vi "Set Wheel Parameter by Name.vi"(8 "error in (no error)":errorcluster, 9 "parameter value":variant, 10 "parameter name":string, 11 "wheel in":refnum<class "NI_Robotics_Wheel.lvclass">) -> (0 "error out":errorcluster, 1 "set?":bool, 3 "wheel out":refnum<class "NI_Robotics_Wheel.lvclass">)   [LabVIEW 2017, in "NI_Robotics_Wheel.lvclass"]
uses:
  <vilib>/robotics/Steering/Wheel/NI_Robotics_Wheel.lvclass
  <vilib>/robotics/Steering/Wheel/NI_Robotics_Wheel.lvclass/NI_Robotics_Wheel.ctl
  <vilib>/robotics/Steering/Wheel/Rotation Direction.ctl
  <vilib>/robotics/Actuation/Motor Communication/NI_Robotics_Motor Communication.lvclass
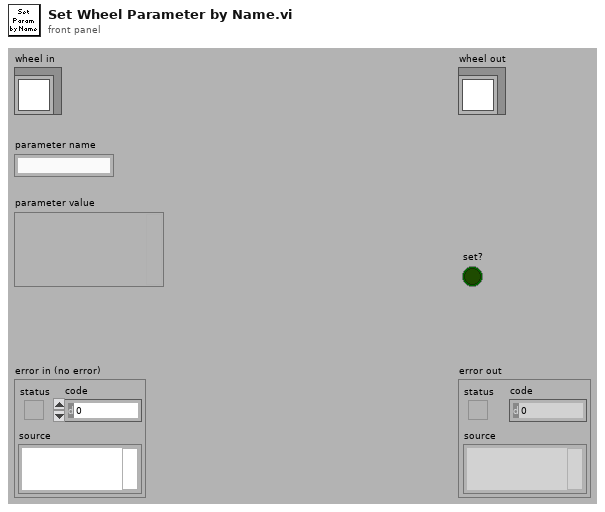
[diagram p1: front panel]
types:
  T1 = typedef "NI_Robotics_Wheel.lvclass/Rotation Direction.ctl" = u16
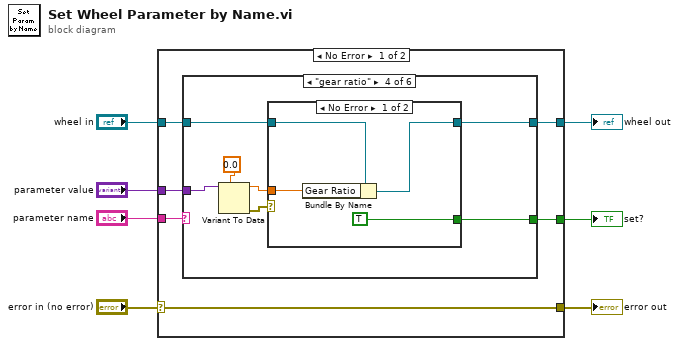
[diagram p0: block diagram]
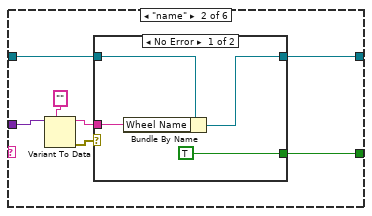
[diagram p3: hidden frame]
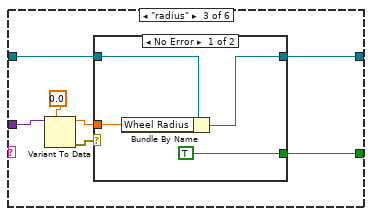
[diagram p5: hidden frame]
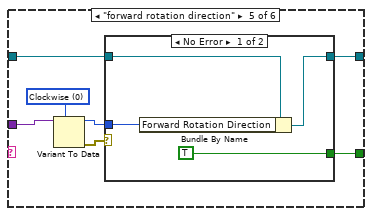
[diagram p8: hidden frame]
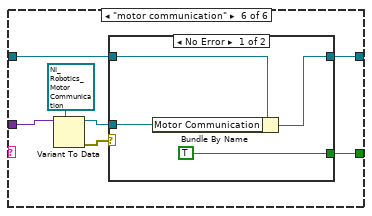
[diagram p10: hidden frame]
diagram:
  n1 = case shown="No Error" "error in (no error)" {
    selector: "error in (no error)" -> [w8 w76]
    tunnel: [w8 w76] -> w6
    tunnel: [w11 w75] -> w4
    tunnel: "wheel in" -> [w13 w75]
    tunnel: "parameter name" -> [w12 _]
    tunnel: "parameter value" -> [w10 _]
    tunnel: [w9 _] -> w1
    frame No Error {
      n2 = case shown="\"gear ratio\"" w12 {
        tunnel: w13 -> [w14 w17 w29 w41 w54 w66]
        tunnel: [w14 w16 w28 w40 w53 w65] -> w11
        tunnel: w10 -> [_ w21 w33 w45 w57 w69]
        tunnel: [_ w15 w27 w39 w52 w64] -> w9
        frame Default {
        }
        frame "name" {
          n3 = Variant To Data(type="", Variant=w21) -> (data=w18:string, error out=w19:errorcluster)  [unwired: 1 in]
          n4 = case shown="No Error" w19 {
            tunnel: w18 -> [w24 _]
            tunnel: w17 -> [w25 w26]
            tunnel: [w23 w26] -> w16
            tunnel: [TRUE _] -> w15
            frame No Error {
              n5 = Bundle By Name(cluster=w25, "Wheel Name"=w24) -> (w23:refnum<class "NI_Robotics_Wheel.lvclass">)
            }
            frame Error {
            }
          }
        }
        frame "radius" {
          n6 = Variant To Data(type=0.0, Variant=w33) -> (data=w30:dbl, error out=w31:errorcluster)  [unwired: 1 in]
          n7 = case shown="No Error" w31 {
            tunnel: w30 -> [w36 _]
            tunnel: w29 -> [w37 w38]
            tunnel: [w35 w38] -> w28
            tunnel: [TRUE _] -> w27
            frame No Error {
              n8 = Bundle By Name(cluster=w37, "Wheel Radius"=w36) -> (w35:refnum<class "NI_Robotics_Wheel.lvclass">)
            }
            frame Error {
            }
          }
        }
        frame "gear ratio" {
          n9 = Variant To Data(type=0.0, Variant=w45) -> (data=w42:dbl, error out=w43:errorcluster)  [unwired: 1 in]
          n10 = case shown="No Error" w43 {
            tunnel: w42 -> [w48 _]
            tunnel: w41 -> [w49 w50]
            tunnel: [w47 w50] -> w40
            tunnel: [TRUE _] -> w39
            frame No Error {
              n11 = Bundle By Name(cluster=w49, "Gear Ratio"=w48) -> (w47:refnum<class "NI_Robotics_Wheel.lvclass">)
            }
            frame Error {
            }
          }
        }
        frame "forward rotation direction" {
          w51 = T1 0 items=["Clockwise", "Counterclockwise"] ("Forward Rotation Direction")
          n12 = Variant To Data(type=w51, Variant=w57) -> (data=w55:T1, error out=w56:errorcluster)  [unwired: 1 in]
          n13 = case shown="No Error" w56 {
            tunnel: w55 -> [w58 _]
            tunnel: w54 -> [w61 w62]
            tunnel: [w60 w62] -> w53
            tunnel: [TRUE _] -> w52
            frame No Error {
              n14 = Bundle By Name(cluster=w61, "Forward Rotation Direction"=w58) -> (w60:refnum<class "NI_Robotics_Wheel.lvclass">)
            }
            frame Error {
            }
          }
        }
        frame "motor communication" {
          n15 = Variant To Data(type=refnum<class "NI_Robotics_Motor Communication.lvclass"> refnum ("Motor Communication"), Variant=w69) -> (data=w67:refnum<class "NI_Robotics_Motor Communication.lvclass">, error out=w68:errorcluster)  [unwired: 1 in]
          n16 = case shown="No Error" w68 {
            tunnel: w67 -> [w70 _]
            tunnel: w66 -> [w73 w74]
            tunnel: [w72 w74] -> w65
            tunnel: [TRUE _] -> w64
            frame No Error {
              n17 = Bundle By Name(cluster=w73, "Motor Communication"=w70) -> (w72:refnum<class "NI_Robotics_Wheel.lvclass">)
            }
            frame Error {
            }
          }
        }
      }
    }
    frame Error {
    }
  }
  "error out" <- w6
  "wheel out" <- w4
  "set?" <- w1
